vi "myRIO_Gil_RT__randomizeMinMax__v3,0.vi"(9 "Input_Increment":u16=1 step=1, 10 "Input_Min":u16=1 step=1, 11 "Input_Max":u16=1 step=1) -> (3 "Output":u16)   [LabVIEW 2014]
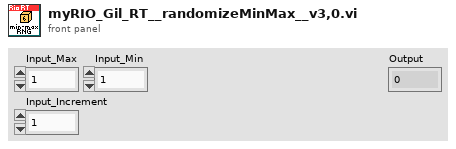
[diagram p1: front panel]
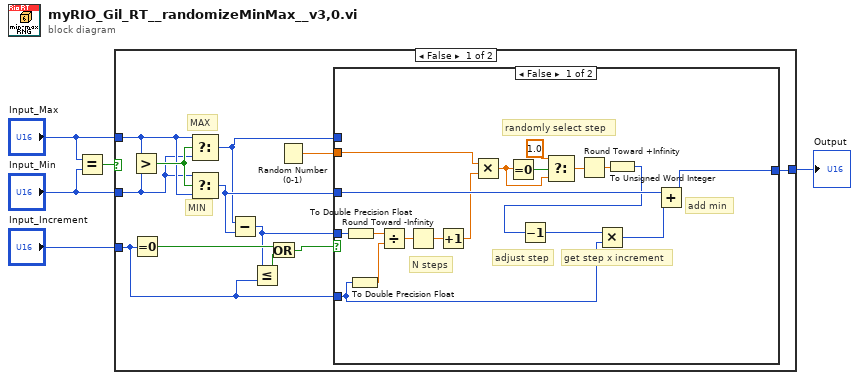
[diagram p0: block diagram]
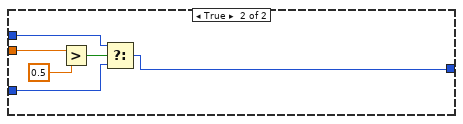
[diagram p2: hidden frame]
diagram:
  n1 = Equal?(x="Input_Max", y="Input_Min") -> (x = y?=w3:bool)
  n2 = case shown="False" w3 {
    tunnel: "Input_Max" -> [w15 w42]
    tunnel: "Input_Min" -> [w14 _]
    tunnel: [w17 w42] -> w5
    tunnel: "Input_Increment" -> [w11 _]
    frame False {
      # "MIN"
      # "MAX"
      n3 = Greater?(x=w15, y=w14) -> (0:w16:bool)
      n4 = Equal To 0?(x=w11) -> (x = 0?=w9:bool)
      n5 = Select(t=w15, s=w16, f=w14) -> (s? t:f=w12:u16)
      n6 = Select(t=w14, s=w16, f=w15) -> (s? t:f=w13:u16)
      n7 = Subtract(x=w12, y=w13) -> (x-y=w6:u16)
      n8 = Less Or Equal?(x=w6, y=w11) -> (x <= y?=w10:bool)
      n9 = Or(x=w9, y=w10) -> (x .or. y?=w8:bool)
      n10 = Random Number (0-1)() -> (number: 0 to 1=w7:dbl)
      n11 = case shown="False" w8 {
        tunnel: w12 -> [_ w39]
        tunnel: w13 -> [w27 w38]
        tunnel: [w26 w37] -> w17
        tunnel: w11 -> [w29 _]
        tunnel: w7 -> [w31 w36]
        tunnel: w6 -> [w35 _]
        frame False {
          # "add min"
          # "get step x increment"
          # "adjust step"
          # "randomly select step"
          # "N steps"
          n12 = To Double Precision Float(number=w35) -> (double precision float=w34:dbl)
          n13 = To Double Precision Float(number=w29) -> (double precision float=w33:dbl)
          n14 = Divide(x=w34, y=w33) -> (x/y=w32:dbl)
          n15 = Round Toward -Infinity(1:w32) -> (0:w25:dbl)
          n16 = Increment(x=w25) -> (x+1=w24:dbl)
          n17 = Multiply(x=w31, y=w24) -> (x*y=w22:dbl)
          n18 = Equal To 0?(x=w22) -> (x = 0?=w23:bool)
          n19 = Select(t=1.0, s=w23, f=w22) -> (s? t:f=w20:dbl)
          n20 = Round Toward +Infinity(x=w20) -> (ceil(x): smallest int >= x=w30:dbl)
          n21 = To Unsigned Word Integer(number=w30) -> (unsigned 16bit integer=w19:u16)
          n22 = Decrement(x=w19) -> (x-1=w18:u16)
          n23 = Multiply(x=w18, y=w29) -> (x*y=w28:u16)
          n24 = Add(x=w27, y=w28) -> (x+y=w26:u16)
        }
        frame True {
          n25 = Greater?(x=w36, y=0.5) -> (0:w40:bool)
          n26 = Select(t=w39, s=w40, f=w38) -> (s? t:f=w37:u16)
        }
      }
    }
    frame True {
    }
  }
  "Output" <- w5
